vi "PDarray.vi"() -> ()   [LabVIEW 2017]
uses:
  <vilib>/DAQmx/read.llb/DAQmx Read (Analog DBL 1Chan 1Samp).vi
  <vilib>/DAQmx/miscellaneous.llb/DAQmx Fill In Error Info.vi
panel:
  out "Numeric 2":dbl
  out "Numeric":dbl
  out "Waveform Chart":cluster{"data":dbl, "data":dbl}(graph)
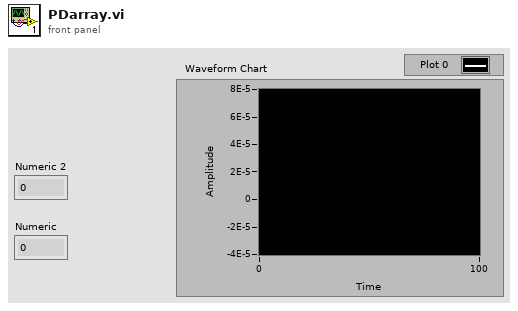
[diagram p1: front panel]
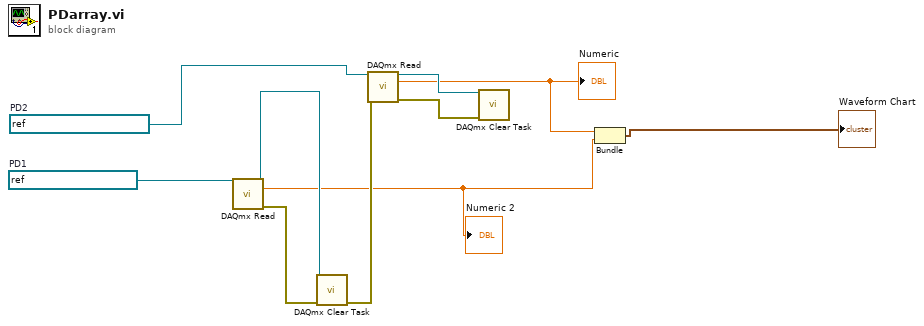
[diagram p0: block diagram]
diagram:
  w9 = refnum<k21> "MyVoltageChannel_1"  # PD2
  w10 = refnum<k21> "MyVoltageChannel"  # PD1
  n1 = call-poly <vilib>:"DAQmx Read.vi"("task/channels in"=w10) -> ("task out"=w5:refnum<k21>, "data"=w2:dbl, "error out"=w6:errorcluster)  [unwired: 12 in]
  "Numeric 2" <- w2
  n2 = call <vilib>:"DAQmx Clear Task.vi"("task in"=w5, "error in"=w6) -> ("error out"=w4:errorcluster)  [unwired: 13 in]
  n3 = call-poly <vilib>:"DAQmx Read.vi"("task/channels in"=w9, "error in"=w4) -> ("task out"=w8:refnum<k21>, "data"=w1:dbl, "error out"=w3:errorcluster)  [unwired: 11 in]
  "Numeric" <- w1
  n4 = call <vilib>:"DAQmx Clear Task.vi"("task in"=w8, "error in"=w3) -> ()  [unwired: 13 in, 1 out]
  n5 = Bundle("data"=w1, "data"=w2) -> (→"Waveform Chart":cluster{"data":dbl, "data":dbl})  [unwired: 1 in]
